vi "Write.vi"(8 "error in (no error)":errorcluster, 10 "Message":string, 11 "TCP_Client in":refnum<class "TCP_Client.lvclass">) -> (0 "error out":errorcluster, 3 "TCP_Client out":refnum<class "TCP_Client.lvclass">)   [LabVIEW 2018, in "TCP_Client.lvlib" / "TCP_Client.lvclass"]
uses:
  TCP_Client.lvclass
  TCP_Client.lvclass/TCP_Client.ctl
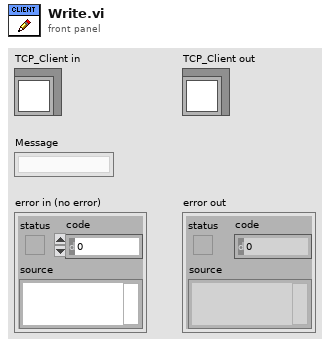
[diagram p1: front panel]
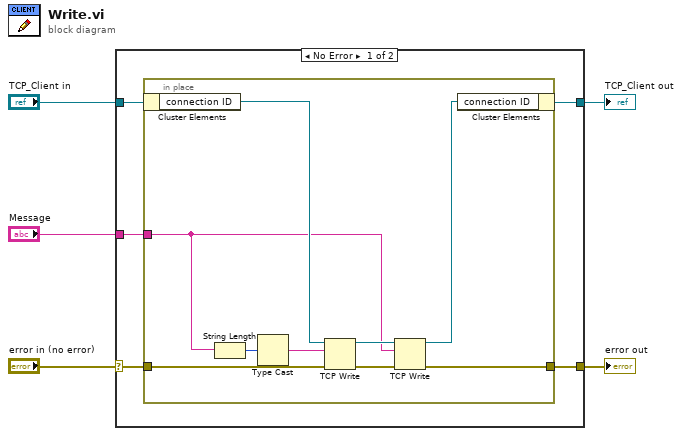
[diagram p0: block diagram]
diagram:
  n1 = case shown="No Error" "error in (no error)" {
    selector: "error in (no error)" -> [w9 w21]
    tunnel: [w7 w21] -> w4
    tunnel: [w6 w20] -> w2
    tunnel: "TCP_Client in" -> [w10 w20]
    tunnel: "Message" -> [w8 _]
    frame No Error {
      n2 = in-place {
        in-place-border: w9 -> [w15]
        in-place-border: w8 -> [w12]
        in-place-border: [w11] -> w7
        n3 = in-place-cluster #1(w10) -> ("connection ID"=w14:refnum<k5>)
        n4 = String Length(string=w12) -> (length=w17:i32)
        n5 = Type Cast(x=w17) -> (*(type *) &x=w16:string)  [unwired: 1 out]
        n6 = TCP Write(connection ID=w14, data in=w16, error in (no error)=w15) -> (connection ID out=w19:refnum<k5>, error out=w18:errorcluster)  [unwired: 2 out]
        n7 = TCP Write(connection ID=w19, data in=w12, error in (no error)=w18) -> (connection ID out=w13:refnum<k5>, error out=w11:errorcluster)  [unwired: 2 out]
        n8 = in-place-cluster #1("connection ID"=w13) -> (w6:refnum<class "TCP_Client.lvclass">)
      }
    }
    frame Error {
    }
  }
  "error out" <- w4
  "TCP_Client out" <- w2
